vi "wsMsgCounter.vi"(11 "Action":enum16{"Increment", "Reset"}(ring)) -> (3 "msgCounter":string)   [LabVIEW 2018, in "HASS-LV-WS_integration.lvlib"]
uses:
  HASS-LV-WS_integration.lvlib
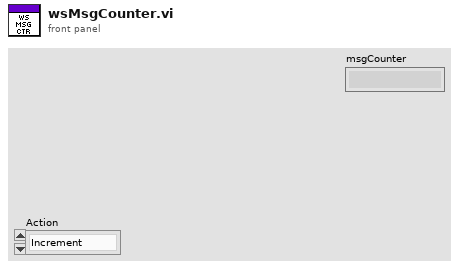
[diagram p1: front panel]
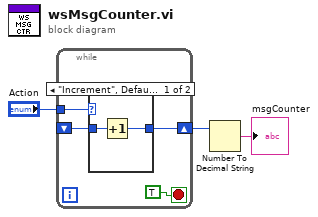
[diagram p0: block diagram]
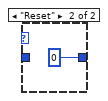
[diagram p2: hidden frame]
diagram:
  n1 = while {
    tunnel: "Action" -> [w6]
    shift-right: [w5] -> w2
    shift-left: _ -> [w4]
    stop <- TRUE stop-if-true
    n2 = case shown="\"Increment\", Default" w6 {
      tunnel: [w8 0] -> w5
      tunnel: w4 -> [w9 _]
      frame "Increment", Default {
        n3 = Increment(x=w9) -> (x+1=w8:i32)
      }
      frame "Reset" {
      }
    }
  }
  n4 = Number To Decimal String(number=w2) -> (decimal integer string=→"msgCounter":string)  [unwired: 1 in]
